vi "Disable Numerics using Xcontrol.vi"() -> ()   [LabVIEW 2012]
uses:
  XControl.xctl
panel:
  out "Boolean 2":bool
  in  "Boolean":bool
  out "Numeric Indicator 3":dbl
  out "Numeric Indicator":dbl
  in  "XControl":T1(xcontrol)
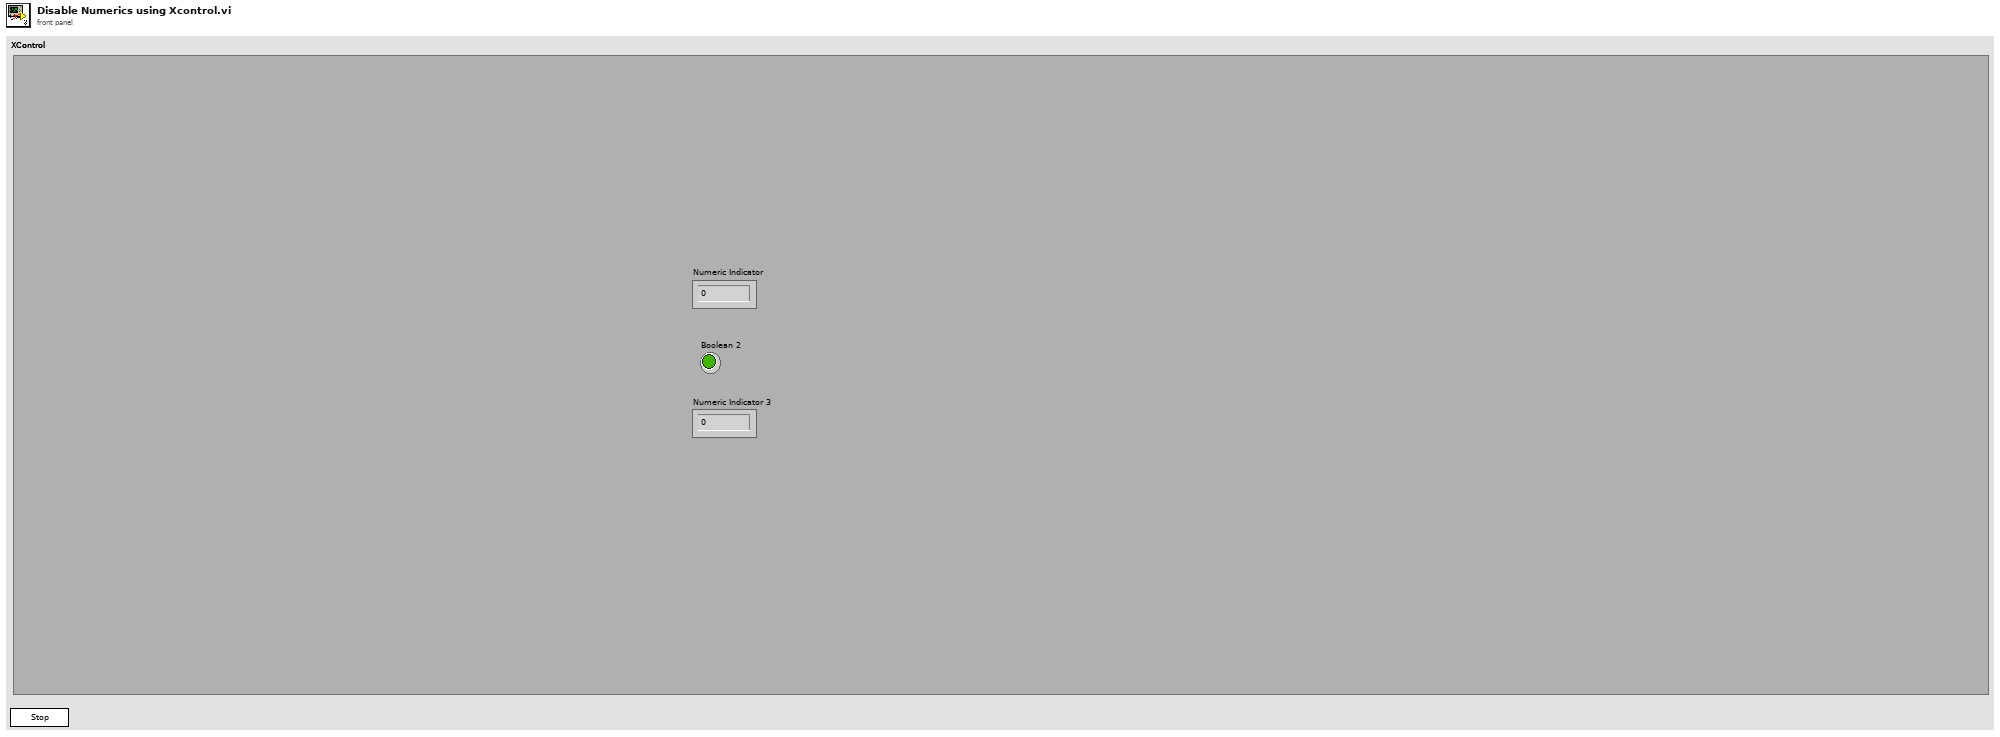
[diagram p1: front panel]
types:
  T1 = cluster{"Ring 10":u8, "Ring 11":u8, "Ring 13":u8, "Ring 14":u8, "Ring 15":u8, "Ring 12":u8, "Ring 16":u8, "Ring 17":u8, "Ring 18":u8, "Ring 19":u8, "Ring 20":u8, "Ring 21":u8, "Ring 22":u8, "Ring 23":u8, "Ring 24":u8, "Ring 25":u8, "Enable":bool, "String 2":string, "String 2":string, "String 3":string, "String 4":string, "String 5":string, "String 6":string, "String 7":string, "String 8":string, "String 9":string, "String 10":string, "String 11":string, "String 12":string, "String 13":string, "String 14":string, "String 15":string, "String 16":string}
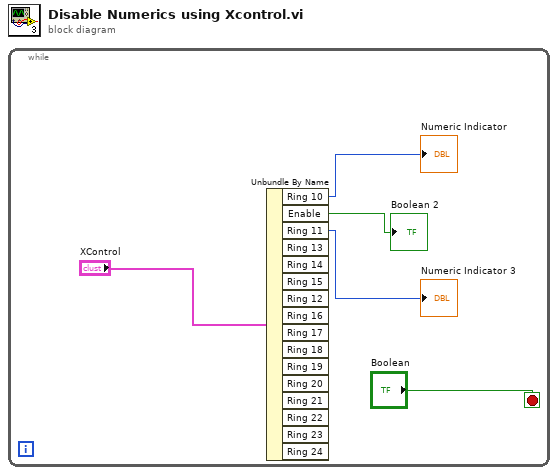
[diagram p0: block diagram]
diagram:
  n1 = while {
    stop <- "Boolean" stop-if-true
    n2 = Unbundle By Name("XControl") -> ("Ring 10"=→"Numeric Indicator":u8, "Enable"=→"Boolean 2":bool, "Ring 11"=→"Numeric Indicator 3":u8)  [unwired: 13 out]
  }
